vi "Producer:Consumer_Variant.vi"() -> ()   [LabVIEW 2023]
panel:
  out "평가 데이터":string
  out "분석 데이터":bool
  out "측정 데이터":i32[](array[numeric])
  in  "종료":bool
  in  "평가":bool
  in  "분석":bool
  in  "측정":bool
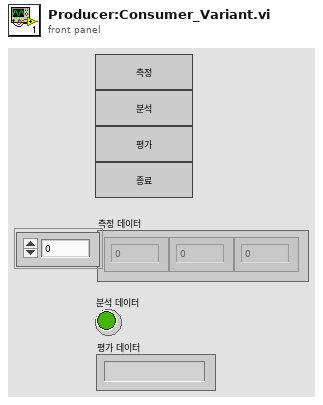
[diagram p1: front panel]
types:
  T1 = typedef "상태.ctl" = enum16{"측정", "분석", "평가", "종료"}
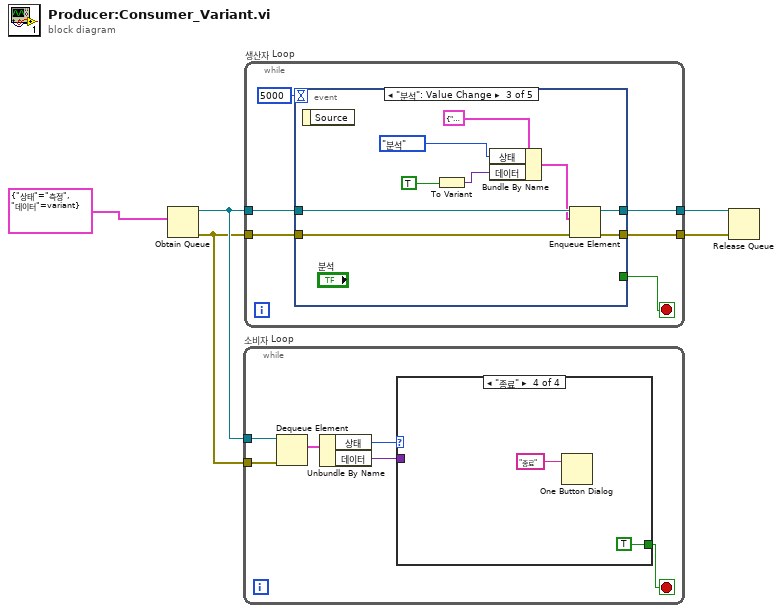
[diagram p0: block diagram]
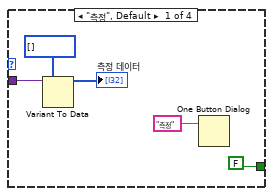
[diagram p2: hidden frame]
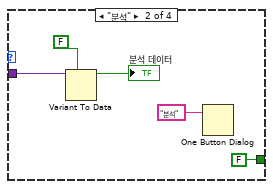
[diagram p3: hidden frame]
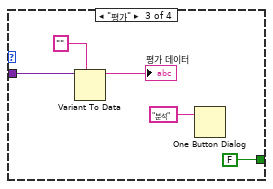
[diagram p4: hidden frame]
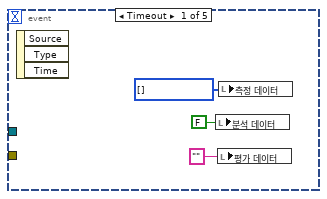
[diagram p5: hidden frame]
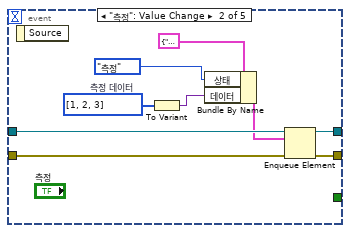
[diagram p6: hidden frame]
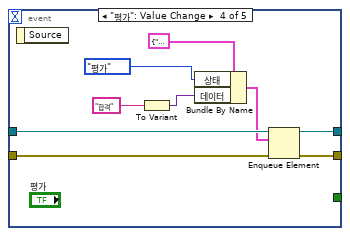
[diagram p7: hidden frame]
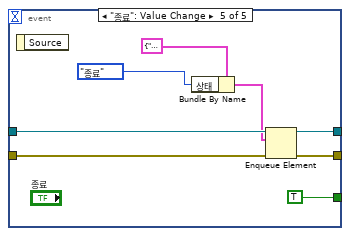
[diagram p8: hidden frame]
diagram:
  n1 = Obtain Queue(element data type=cluster{"상태":T1, "데이터":variant} {"상태"=enum."측정", "데이터"=variant}) -> (queue out=w3:refnum<queue>, error out=w2:errorcluster)  [unwired: 4 in, 1 out]
  n2 = while "소비자 Loop" {
    tunnel: w3 -> [w11]
    tunnel: w2 -> [w10]
    stop <- w6 stop-if-true
    n3 = Dequeue Element(queue=w11, error in (no error)=w10) -> (element=w9:cluster{"상태":T1, "데이터":variant})  [unwired: 1 in, 3 out]
    n4 = Unbundle By Name(w9) -> ("상태"=w8:T1, "데이터"=w7:variant)
    n5 = case shown="\"종료\"" w8 {
      tunnel: w7 -> [w16 w21 w25 _]
      tunnel: [FALSE FALSE FALSE TRUE] -> w6
      frame "측정", Default {
        n6 = Variant To Data(type=i32[] [] ("측정 데이터"), Variant=w16) -> (data=→"측정 데이터":i32[])  [unwired: 1 in, 1 out]
        n7 = One Button Dialog(message="측정") -> ()  [unwired: 1 in, 1 out]
      }
      frame "분석" {
        n8 = Variant To Data(type=FALSE ("분석 데이터"), Variant=w21) -> (data=→"분석 데이터":bool)  [unwired: 1 in, 1 out]
        n9 = One Button Dialog(message="분석") -> ()  [unwired: 1 in, 1 out]
      }
      frame "평가" {
        n10 = Variant To Data(type="" ("평가 데이터"), Variant=w25) -> (data=→"평가 데이터":string)  [unwired: 1 in, 1 out]
        n11 = One Button Dialog(message="분석") -> ()  [unwired: 1 in, 1 out]
      }
      frame "종료" {
        n12 = One Button Dialog(message="종료") -> ()  [unwired: 1 in, 1 out]
      }
    }
  }
  n13 = while "생산자 Loop" {
    tunnel: w2 -> [w34]
    tunnel: [w33] -> w5
    tunnel: w3 -> [w32]
    tunnel: [w31] -> w4
    stop <- w30 stop-if-true
    n14 = event shown="[2] \"분석\": Value Change" {
      selector: _ -> [_ _ _ _ _]
      dyn-events: _ -> [_ _ _ _ _]
      timeout: 5000 -> [_ _ _ _ _]
      tunnel: w34 -> [_ w46 w49 w62 w68]
      tunnel: [_ w45 w50 w61 w67] -> w33
      tunnel: w32 -> [_ w44 w52 w64 w70]
      tunnel: [_ w43 w51 w63 w69] -> w31
      tunnel: [_ _ _ _ TRUE] -> w30
      event Timeout {
        n15 = event-data() -> ()  [unwired: 1 in, 3 out]
        n16 = local write "분석 데이터"(FALSE ("분석 데이터")) -> ()
        n17 = local write "평가 데이터"("" ("평가 데이터")) -> ()
        n18 = local write "측정 데이터"(i32[] [] ("측정 데이터")) -> ()
      }
      event "측정": Value Change {
        w39 = i32[] [1, 2, 3]  # 측정 데이터
        n19 = event-data() -> ()  [unwired: 1 in, 1 out]
        n20 = To Variant(anything=w39) -> (Variant=w40:variant)
        n21 = Bundle By Name(cluster=cluster{"상태":T1, "데이터":variant} {"상태"=enum."측정", "데이터"=variant}, "상태"=상태."측정", "데이터"=w40) -> (w38:cluster{"상태":T1, "데이터":variant})
        n22 = Enqueue Element(queue=w44, element=w38, error in (no error)=w46) -> (queue out=w43:refnum<queue>, error out=w45:errorcluster)  [unwired: 1 in, 1 out]
      }
      event "분석": Value Change {
        n23 = event-data() -> ()  [unwired: 1 in, 1 out]
        n24 = To Variant(anything=TRUE ("분석 데이터")) -> (Variant=w53:variant)
        n25 = Bundle By Name(cluster=cluster{"상태":T1, "데이터":variant} {"상태"=enum."측정", "데이터"=variant}, "상태"=상태."분석", "데이터"=w53) -> (w47:cluster{"상태":T1, "데이터":variant})
        n26 = Enqueue Element(queue=w52, element=w47, error in (no error)=w49) -> (queue out=w51:refnum<queue>, error out=w50:errorcluster)  [unwired: 1 in, 1 out]
      }
      event "평가": Value Change {
        n27 = event-data() -> ()  [unwired: 1 in, 1 out]
        n28 = To Variant(anything="합격" ("평가 데이터")) -> (Variant=w58:variant)
        n29 = Bundle By Name(cluster=cluster{"상태":T1, "데이터":variant} {"상태"=enum."측정", "데이터"=variant}, "상태"=상태."평가", "데이터"=w58) -> (w57:cluster{"상태":T1, "데이터":variant})
        n30 = Enqueue Element(queue=w64, element=w57, error in (no error)=w62) -> (queue out=w63:refnum<queue>, error out=w61:errorcluster)  [unwired: 1 in, 1 out]
      }
      event "종료": Value Change {
        n31 = event-data() -> ()  [unwired: 1 in, 1 out]
        n32 = Bundle By Name(cluster=cluster{"상태":T1, "데이터":variant} {"상태"=enum."측정", "데이터"=variant}, "상태"=상태."종료") -> (w66:cluster{"상태":T1, "데이터":variant})
        n33 = Enqueue Element(queue=w70, element=w66, error in (no error)=w68) -> (queue out=w69:refnum<queue>, error out=w67:errorcluster)  [unwired: 1 in, 1 out]
      }
    }
  }
  n34 = Release Queue(queue=w4, error in (no error)=w5) -> ()  [unwired: 1 in, 3 out]
